vi "PH_AxisGUI_NF2.set i Attr.vi"(2 "error in (no error)":errorcluster, 3 "DB Entry to read":string) -> (0 "error out":errorcluster, 1 "i Attributes":T1={"GUI Refs"={"Delete"=refnum, "Instance Status"=refnum, "Width Axis 1"=refnum, "Width Axis 2"=refnum}, "Instance"="N/A", "System"="N/A", "Width Axis 1"=0, "Width Axis 2"=0, "Sign Change Axis 1"=FALSE, "Sign Change Axis 2"=FALSE, "Motor Axis 1"=0, "Motor Axis 2"=0})   [LabVIEW 2014, in "PH_AxisGUI_NF2.lvlib"]
doc: "This VI reads the DB entries and sets several attributes and GUI element settings."
uses:
  PH_AxisGUI_NF2.lvlib
  PH_AxisGUI_NF2.i attribute.ctl
  PH_Basics/PH_Common/PH_Common.lvlib
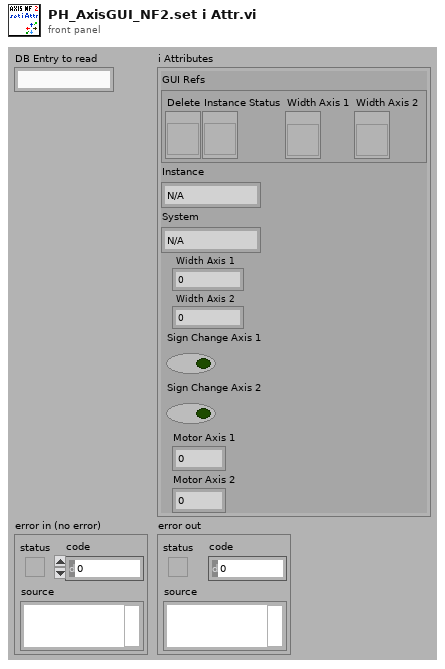
[diagram p1: front panel]
types:
  T1 = typedef "PH_AxisGUI_NF2.lvlib/PH_AxisGUI_NF2.i attribute.ctl" = cluster{"GUI Refs":cluster{"Delete":refnum<vi>, "Instance Status":refnum<vi>, "Width Axis 1":refnum<vi>, "Width Axis 2":refnum<vi>}, "Instance":string, "System":string, "Width Axis 1":i32, "Width Axis 2":i32, "Sign Change Axis 1":bool, "Sign Change Axis 2":bool, "Motor Axis 1":i32, "Motor Axis 2":i32}
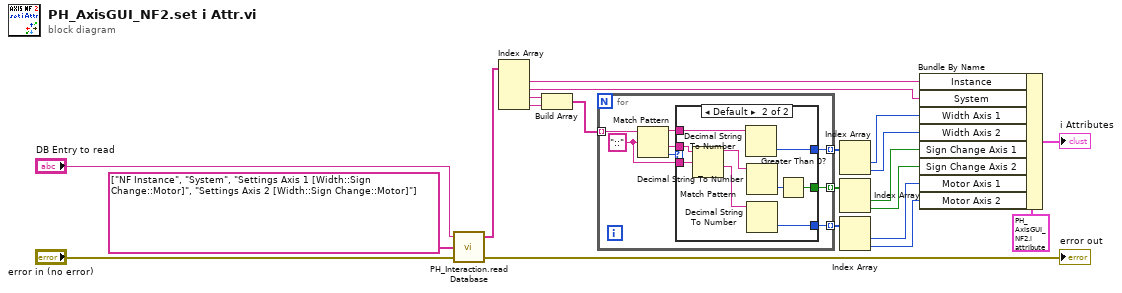
[diagram p0: block diagram]
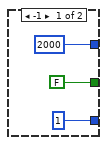
[diagram p2: hidden frame]
diagram:
  n1 = call "PH_Interaction.read Database.vi"("error in (no error)"="error in (no error)", "Strings to search for"=string[] ["NF Instance", "System", "Settings Axis 1 [Width::Sign Change::Motor]", "Settings Axis 2 [Width::Sign Change::Motor]"], "DB Entry to read"="DB Entry to read") -> ("error out"=→"error out":errorcluster, "Values"=w13:string[])  [unwired: 1 in]
  n2 = Index Array(array=w13) -> (element #1=w21:string, element #2=w20:string, element #3=w12:string, element #4=w10:string)  [unwired: 4 in]
  n3 = Build Array(w12, w10) -> (w11:string[])
  n4 = for {
    tunnel: [w26] -> w18 mode=indexing
    tunnel: [w25] -> w17 mode=indexing
    tunnel: [w24] -> w4 mode=indexing
    tunnel: w11 -> [w22] mode=indexing
    w28 = "::" ("regular expression")
    n5 = Match Pattern(string=w22, regular expression=w28) -> (before substring=w27:string, after substring=w29:string, offset past match=w23:i32)  [unwired: 1 in, 1 out]
    n6 = case shown="Default" w23 {
      tunnel: w29 -> [_ w41]
      tunnel: w28 -> [_ w40]
      tunnel: w27 -> [_ w39]
      tunnel: [2000 w38] -> w26
      tunnel: [FALSE w35] -> w25
      tunnel: [1 w33] -> w24
      frame -1 {
      }
      frame Default {
        n7 = Match Pattern(string=w41, regular expression=w40) -> (before substring=w37:string, after substring=w34:string)  [unwired: 1 in, 2 out]
        n8 = Decimal String To Number(string=w39) -> (number=w38:i32)  [unwired: 2 in, 1 out]
        n9 = Decimal String To Number(string=w37) -> (number=w36:i32)  [unwired: 2 in, 1 out]
        n10 = Decimal String To Number(string=w34) -> (number=w33:i32)  [unwired: 2 in, 1 out]
        n11 = Greater Than 0?(x=w36) -> (x > 0?=w35:bool)
      }
    }
  }
  n12 = Index Array(array=w18) -> (element #1=w9:i32, element #2=w8:i32)  [unwired: 2 in]
  n13 = Index Array(array=w17) -> (element #1=w7:bool, element #2=w6:bool)  [unwired: 2 in]
  n14 = Index Array(array=w4) -> (element #1=w5:i32, element #2=w3:i32)  [unwired: 2 in]
  n15 = Bundle By Name(cluster=T1 {"GUI Refs"={"Delete"=refnum, "Instance Status"=refnum, "Width Axis 1"=refnum, "Width Axis 2"=refnum}, "Instance"="N/A", "System"="N/A", "Width Axis 1"=0, "Width Axis 2"=0, "Sign Change Axis 1"=FALSE, "Sign Change Axis 2"=FALSE, "Motor Axis 1"=0, "Motor Axis 2"=0} ("i attribute"), "Instance"=w21, "System"=w20, "Width Axis 1"=w9, "Width Axis 2"=w8, "Sign Change Axis 1"=w7, "Sign Change Axis 2"=w6, "Motor Axis 1"=w5, "Motor Axis 2"=w3) -> (→"i Attributes":T1)
